vi "eSpinADR112.vi"() -> ()   [LabVIEW 2017]
doc: "This vi interfaces with the ADR112 Serial Board to illuminate a red and green physical led upon certain conditions. The vi generates random numbers from 0 - 100 and if the number is greater than 50 then the electron is a spin up electron, and the red led illuminates. Conversely, if the number is less than 50 then it is spin down and the green led illuminates."
uses:
  <vilib>/Instr/_visa.llb/VISA Configure Serial Port (Instr).vi
panel:
  in  "COM Port":refnum<visa-resource-name>
  out "Total Spin Down":i32
  out "Total Spin Up":i32
  in  "?":bool
  out "Spin Down":bool
  out "Spin Up":bool
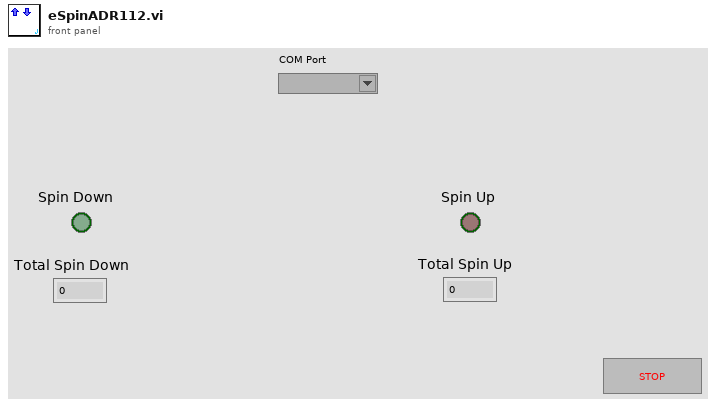
[diagram p1: front panel]
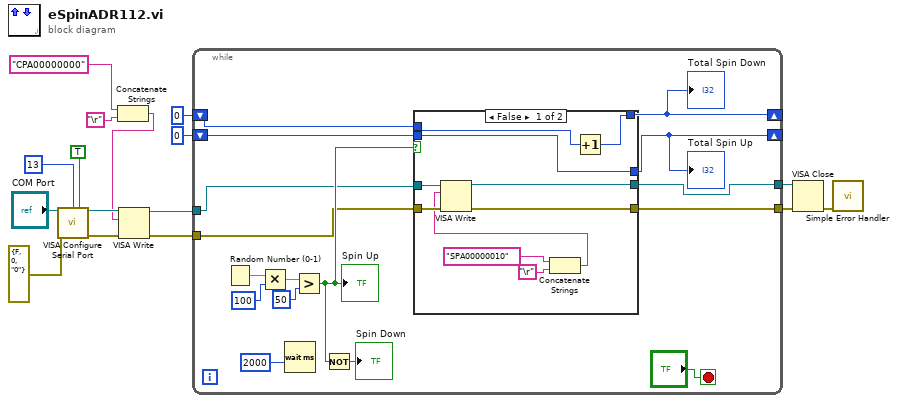
[diagram p0: block diagram]
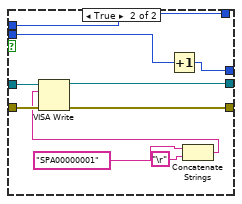
[diagram p2: hidden frame]
diagram:
  n1 = call-poly "VISA Configure Serial Port"("VISA resource name"="COM Port", "termination char\n(0xA = '\\n' = LF)"=u8 13 ("termination char\n(0xA = '\\n' = LF)"), "Enable Termination\nChar (T)"=TRUE ("Enable Termination\nChar (T)"), "error in (no error)"=errorcluster {"status"=FALSE, "code"=0, "source"="0"}) -> ("VISA resource name out"=w6:refnum<visa-resource-name>, "error out"=w7:errorcluster)  [unwired: 10 in]
  n2 = Concatenate Strings("CPA00000000" ("write buffer"), "\r") -> (w1:string)
  n3 = VISA Write(VISA resource name=w6, write buffer=w1, error in (no error)=w7) -> (VISA resource name out=w5:refnum<visa-resource-name>, error out=w4:errorcluster)  [unwired: 1 out]
  n4 = while {
    shift-right: [w21] -> _
    shift-left: 0 -> [w25]
    shift-right: [w22] -> _
    shift-left: 0 -> [w26]
    tunnel: w5 -> [w20]
    tunnel: w4 -> [w19]
    tunnel: [w18] -> w11
    tunnel: [w17] -> w12
    stop <- "?" stop-if-true
    n5 = Random Number (0-1)() -> (number: 0 to 1=w32:dbl)
    n6 = Multiply(x=w32, y=100) -> (x*y=w23:dbl)
    n7 = Wait (ms)(milliseconds to wait=2000) -> ()  [unwired: 1 out]
    n8 = Greater?(x=w23, y=50) -> (0:w27:bool)
    "Spin Up" <- w27
    n9 = Not(x=w27) -> (.not. x?=→"Spin Down":bool)
    n10 = case shown="False" w27 {
      tunnel: w25 -> [w42 w50]
      tunnel: w26 -> [w41 w52]
      tunnel: [w42 w51] -> w21
      tunnel: [w40 w52] -> w22
      tunnel: w20 -> [w38 w48]
      tunnel: w19 -> [w39 w49]
      tunnel: [w37 w47] -> w18
      tunnel: [w36 w46] -> w17
      frame False {
        n11 = Concatenate Strings("SPA00000010", "\r") -> (w33:string)
        n12 = VISA Write(VISA resource name=w38, write buffer=w33, error in (no error)=w39) -> (VISA resource name out=w37:refnum<visa-resource-name>, error out=w36:errorcluster)  [unwired: 1 out]
        n13 = Increment(x=w41) -> (x+1=w40:i32)
      }
      frame True {
        n14 = Increment(x=w50) -> (x+1=w51:i32)
        n15 = Concatenate Strings("SPA00000001", "\r") -> (w43:string)
        n16 = VISA Write(VISA resource name=w48, write buffer=w43, error in (no error)=w49) -> (VISA resource name out=w47:refnum<visa-resource-name>, error out=w46:errorcluster)  [unwired: 1 out]
      }
    }
    "Total Spin Up" <- w21
    "Total Spin Down" <- w22
  }
  n17 = VISA Close(VISA resource name=w11, error in (no error)=w12) -> (error out=w10:errorcluster)
  n18 = call <vilib>:"Simple Error Handler.vi"("error in (no error)"=w10) -> ()  [unwired: 4 in, 5 out]
